vi "Convertor.system.vi"(7 "String":string, 9 "DBL":dbl) -> (0 "String to DBL":dbl, 3 "DBL to string":string)   [LabVIEW 2020]
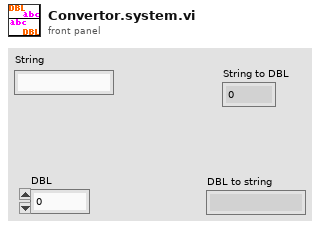
[diagram p1: front panel]
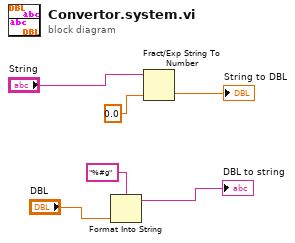
[diagram p0: block diagram]
diagram:
  n1 = Format Into String(format string="%#g", "DBL") -> (resulting string=→"DBL to string":string)  [unwired: 2 in, 1 out]
  n2 = Fract/Exp String To Number(string="String", default (0 dbl)=0.0 ("default (0 DBL)")) -> (number=→"String to DBL":dbl)  [unwired: 2 in, 1 out]
